vi "Set - Matrix - Real.vi"(8 "error in":errorcluster, 9 "value":dbl[][](array[numeric]), 10 "variable name":string, 11 "pipe in":T1) -> (0 "error out":errorcluster, 3 "pipe out":T1)   [LabVIEW 2013, in "GOLPI library.lvlib"]
uses:
  GOLPI library.lvlib
  LV Process.lvlibp/Pipe Handle.ctl
  LV Process.lvlibp
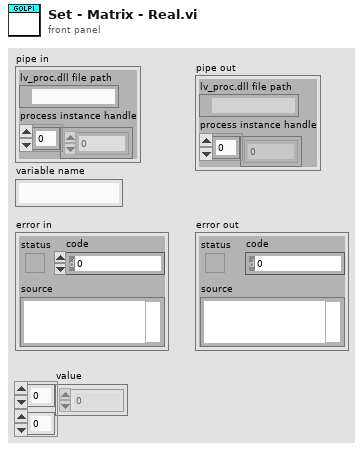
[diagram p1: front panel]
types:
  T1 = typedef "LV Process.lvlibp/Pipe Handle.ctl" = cluster{"lv_proc.dll file path":path, "process instance handle":u32[]}
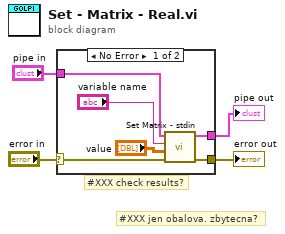
[diagram p0: block diagram]
diagram:
  # "#XXX jen obalova. zbytecna?"
  # "#XXX check results?"
  n1 = case shown="No Error" "error in" {
    selector: "error in" -> [w8 w12]
    tunnel: [w7 w12] -> w4
    tunnel: "pipe in" -> [w6 w11]
    tunnel: [w5 w11] -> w1
    frame No Error {
      n2 = call "Set Matrix - stdin.vi"("error in"=w8, "value"="value", "variable name"="variable name", "pipe in"=w6) -> ("error out"=w7:errorcluster, "pipe out"=w5:T1)  [unwired: 6 in]
    }
    frame Error {
    }
  }
  "error out" <- w4
  "pipe out" <- w1
